vi "Feed.vi"() -> ()   [LabVIEW 2014]
panel:
  in  "닫기":bool
  in  "전송":bool
  in  "Message":string="사용 버전:2.0.0.18\n이름/닉네임:\nE-Mail :\n문의 사항/에러/건의/기타\n내용:" caption="메시지"
  # "개발자에게 피드백"
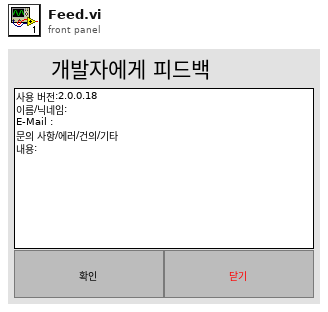
[diagram p1: front panel]
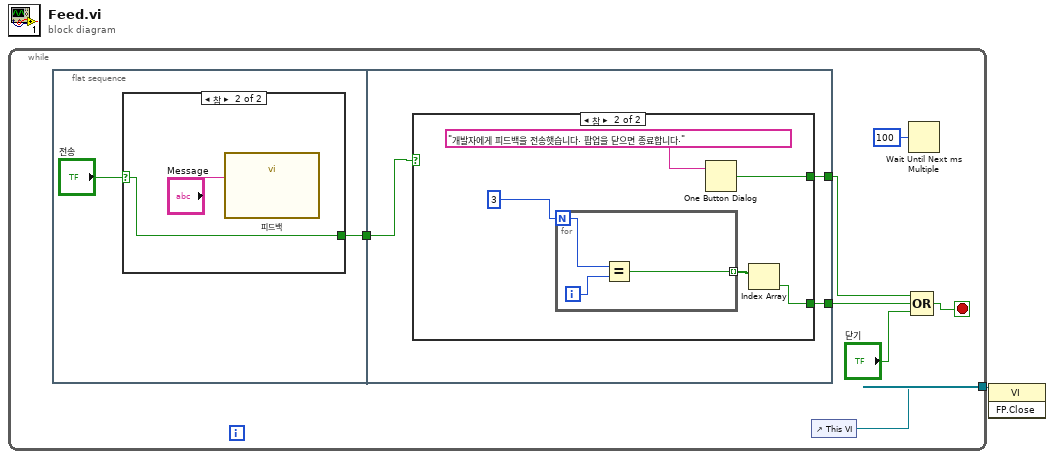
[diagram p0: block diagram]
diagram:
  n1 = while {
    tunnel: [w8] -> w1
    stop <- w3 stop-if-true
    n2 = flat-sequence {
      tunnel: [w9] -> w7
      tunnel: w7 -> [w15]
      tunnel: [w14] -> w4
      tunnel: [w13] -> w5
      frame #0 {
        n3 = case shown="참" "전송" {
          selector: "전송" -> [_ w11]
          tunnel: [_ w11] -> w9
          frame False {
          }
          frame True {
            n4 = call "피드백"("Message"="Message") -> ()  [unwired: 10 in, 1 out]
          }
        }
      }
      frame #1 {
        n5 = case shown="참" w15 {
          tunnel: [_ w19] -> w14
          tunnel: [_ w16] -> w13
          frame False {
          }
          frame True {
            n6 = for {
              N: 3 -> [w22]
              tunnel: [w21] -> w17 mode=indexing
              i -> [w23]
              n7 = Equal?(x=w22, y=w23) -> (x = y?=w21:bool)
            }
            n8 = One Button Dialog(message="개발자에게 피드백을 전송햇습니다. 팝업을 닫으면 종료합니다." ("메시지")) -> (true=w19:bool)  [unwired: 1 in]
            n9 = Index Array(array=w17) -> (element=w16:bool)  [unwired: 1 in]
          }
        }
      }
    }
    n10 = control-ref of="This VI"() -> (w8:refnum<vi>)
    n11 = Wait Until Next ms Multiple(millisecond multiple=u32 100 ("ms 배수")) -> ()  [unwired: 1 out]
    n12 = Compound Arithmetic op=OR(w4, w5, "닫기") -> (w3:bool)
  }
  n13 = invoke class="VI" method="FP.Close"(reference=w1) -> ()  [unwired: 2 in, 3 out]
